vi "Create Notifiers.vi"(8 "error in (no error)":errorcluster) -> (0 "error out":errorcluster, 3 "output cluster":T1)   [LabVIEW 2015]
uses:
  Notifiers.ctl
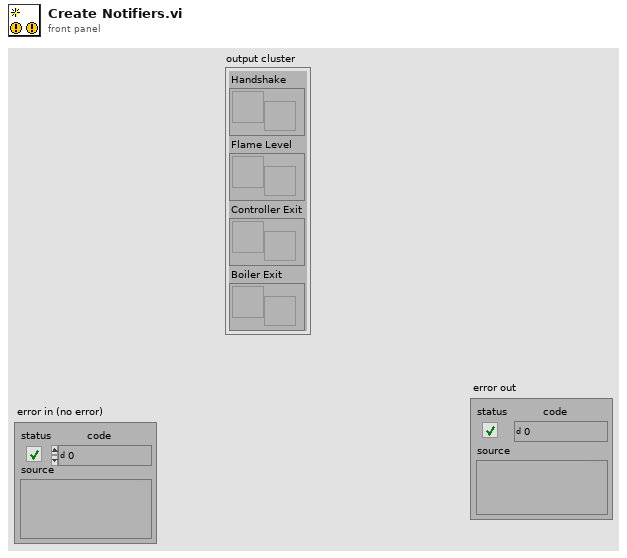
[diagram p1: front panel]
types:
  T1 = typedef "Notifiers.ctl" = cluster{"Handshake":refnum<notifier>, "Flame Level":refnum<notifier>, "Controller Exit":refnum<notifier>, "Boiler Exit":refnum<notifier>}
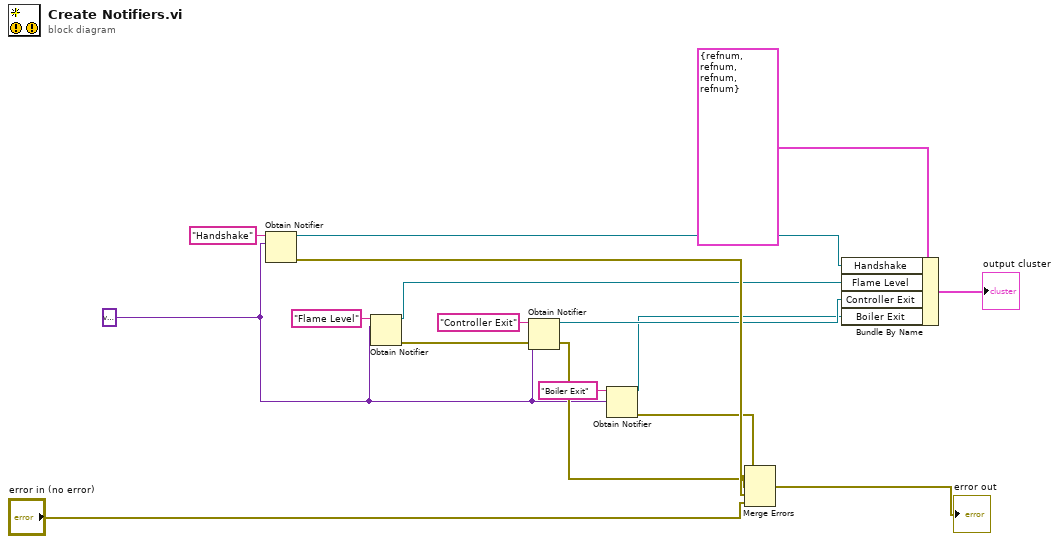
[diagram p0: block diagram]
diagram:
  w7 = variant
  n1 = Obtain Notifier(name (unnamed)="Handshake", notification data type=w7) -> (notifier out=w5:refnum<notifier>, error out=w14:errorcluster)  [unwired: 2 in, 1 out]
  n2 = Obtain Notifier(name (unnamed)="Flame Level", notification data type=w7) -> (notifier out=w3:refnum<notifier>, error out=w13:errorcluster)  [unwired: 2 in, 1 out]
  n3 = Obtain Notifier(name (unnamed)="Controller Exit", notification data type=w7) -> (notifier out=w2:refnum<notifier>)  [unwired: 2 in, 2 out]
  n4 = Obtain Notifier(name (unnamed)="Boiler Exit", notification data type=w7) -> (notifier out=w1:refnum<notifier>, error out=w12:errorcluster)  [unwired: 2 in, 1 out]
  n5 = Merge Errors(w12, w13, w13, w14, "error in (no error)") -> (→"error out":errorcluster)
  n6 = Bundle By Name(cluster=T1 {"Handshake"=refnum, "Flame Level"=refnum, "Controller Exit"=refnum, "Boiler Exit"=refnum}, "Handshake"=w5, "Flame Level"=w3, "Controller Exit"=w2, "Boiler Exit"=w1) -> (→"output cluster":T1)
